vi "Igniter.vi"(8 "Pressure In (psi)":dbl, 9 "Ignition":bool, 10 "Previous Ignition":bool, 11 "Previous Ox Sol":bool) -> (0 "Spark Waveform":waveform(dbl), 2 "Fuel Solenoid":bool, 3 "Ox Solenoid":bool)   [LabVIEW 2016]
uses:
  <vilib>/measure/NI_MABase.lvlib
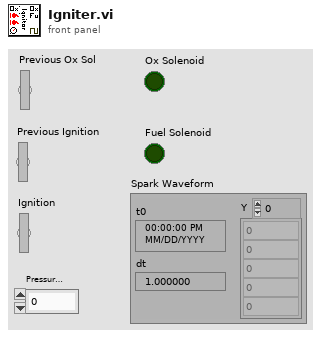
[diagram p1: front panel]
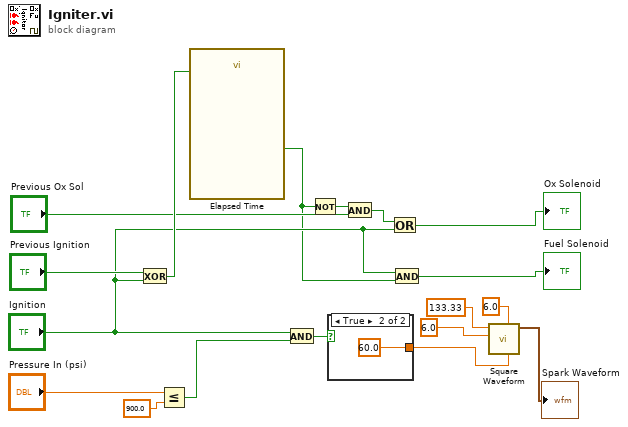
[diagram p0: block diagram]
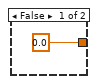
[diagram p2: hidden frame]
diagram:
  n1 = Exclusive Or(1:"Ignition", 2:"Previous Ignition") -> (0:w14:bool)
  n2 = Less Or Equal?(x="Pressure In (psi)", y=900.0) -> (x <= y?=w12:bool)
  n3 = call "Elapsed Time"("Reset"=w14) -> ("Time has Elapsed"=w1:bool)  [unwired: 11 in, 7 out]
  n4 = And(x="Ignition", y=w12) -> (x .and. y?=w5:bool)
  n5 = Not(x=w1) -> (.not. x?=w3:bool)
  n6 = case shown="True" w5 {
    tunnel: [0.0 60.0] -> w8
    frame False {
    }
    frame True {
    }
  }
  n7 = And(x=w3, y="Previous Ox Sol") -> (x .and. y?=w18:bool)
  n8 = Or(x=w18, y="Ignition") -> (x .or. y?=→"Ox Solenoid":bool)
  n9 = And(x="Ignition", y=w1) -> (x .and. y?=→"Fuel Solenoid":bool)
  n10 = call <vilib>:"Square Waveform.vi"("duty cycle (%)"=w8, "offset"=6.0, "amplitude"=6.0, "frequency"=133.33) -> ("signal out"=→"Spark Waveform":waveform(dbl))  [unwired: 6 in, 1 out]
